vi "Manipulate FROG Trace.vi"(8 "error in (no error)":errorcluster caption="entrée d'erreur (pas d'erreur)", 10 "Transpose FROG Trace":bool, 11 "File mainpulate en entrée":refnum<class "File manipulate.lvclass">) -> (0 "error out":errorcluster caption="sortie d'erreur", 1 "Wavelenght_New":dbl[](array[numeric]), 2 "DelayVector":dbl[](array[numeric]), 3 "File mainpulate en sortie":refnum<class "File manipulate.lvclass">, 4 "Data Reshape":dbl[][](array[numeric]), 5 "Data Manipulate FROG TRACE":T1 {"WavelengthPoints_increment" format="%.16f"; "WavelengthPoints_center" format="%#.13g"})   [LabVIEW 2024, in "File manipulate.lvclass"]
uses:
  File manipulate.lvclass
  Data Manipulate FROG TRACE.ctl
  FROG Trace -Etat.ctl
  File manipulate.lvclass/File manipulate.ctl
  <userlib>/_Hooovahh/Array VIMs/Controls/Enum - Rows Columns.ctl
  <vilib>/Analysis/1siggen.llb/Ramp Pattern by Samples.vi
  6a061561-2aec-49c3-b07e-13be07ae40b1.vi
  d13b3189-b418-4897-bbe3-08cafe995864.vi
  <vilib>/Analysis/baseanly.llb/Mean (DBL).vi
  <vilib>/gmath/interp.llb/Interpolate 2D (1d xi,yi).vi
  <vilib>/Analysis/NI_AALBase.lvlib
  <vilib>/gmath/NI_Gmath.lvlib
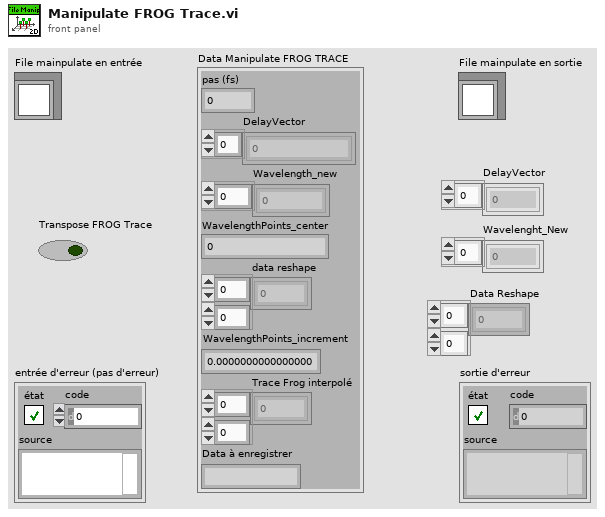
[diagram p1: front panel]
types:
  T1 = typedef "File manipulate.lvclass/Data Manipulate FROG TRACE.ctl" = cluster{"pas (fs)":ext, "DelayVector":dbl[], "Wavelength_new":dbl[], "WavelengthPoints_center":dbl, "data reshape":dbl[][], "WavelengthPoints_increment":dbl, "Trace Frog interpolé":dbl[][], "Data à enregistrer":string}
  T2 = typedef "File manipulate.lvclass/FROG Trace -Etat.ctl" = enum16{"Conversion Pas um to fs", "Delay Vector", "Reshape FROG Trace", "Wavelenght New", "Wavelenght Center", "Wavelenght Point increment", "Interpolation 2D", "Concaner en txt", "Enregistrement"}
  T3 = typedef "Enum - Rows Columns.ctl" = enum16{"Rows", "Columns"}
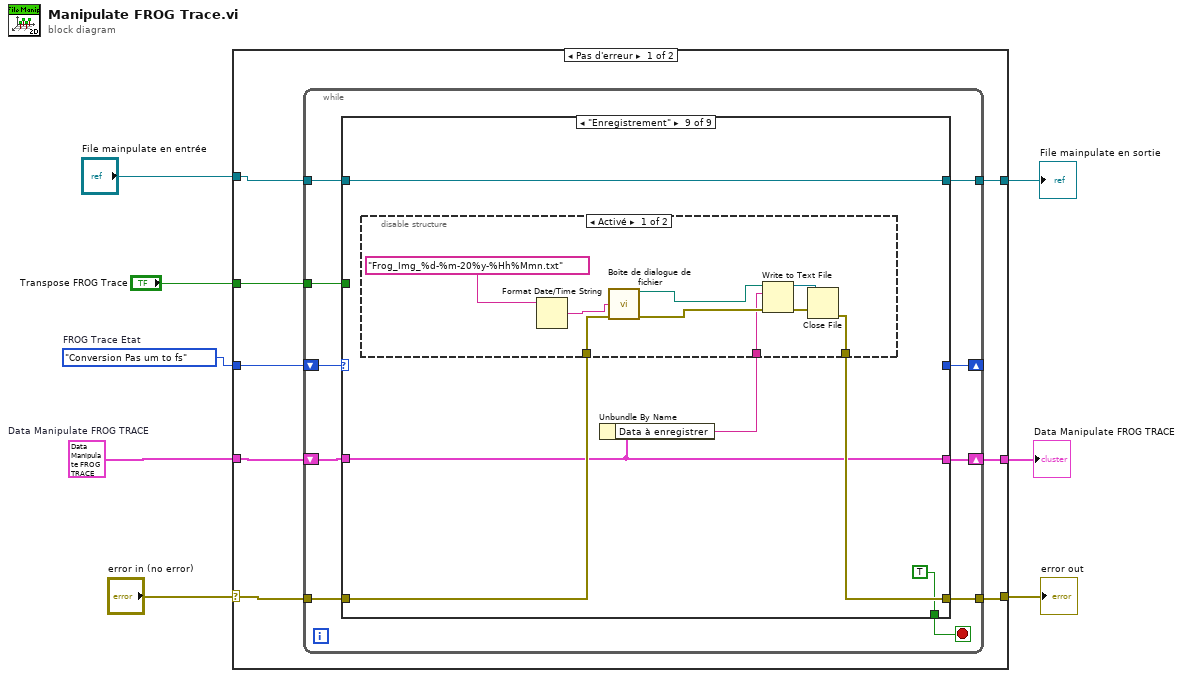
[diagram p0: block diagram]
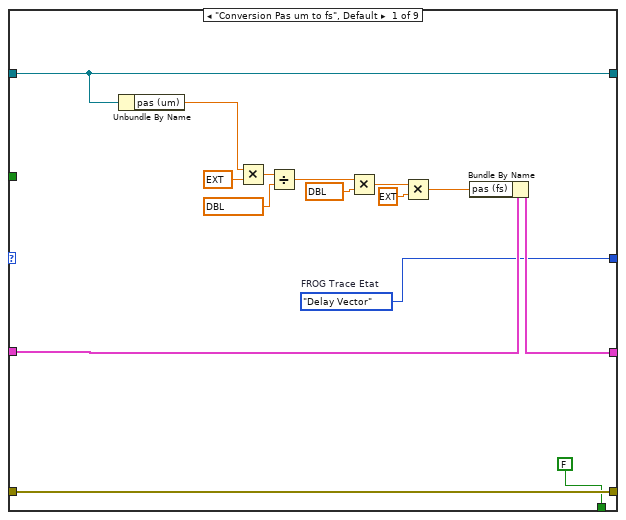
[diagram p2: hidden frame]
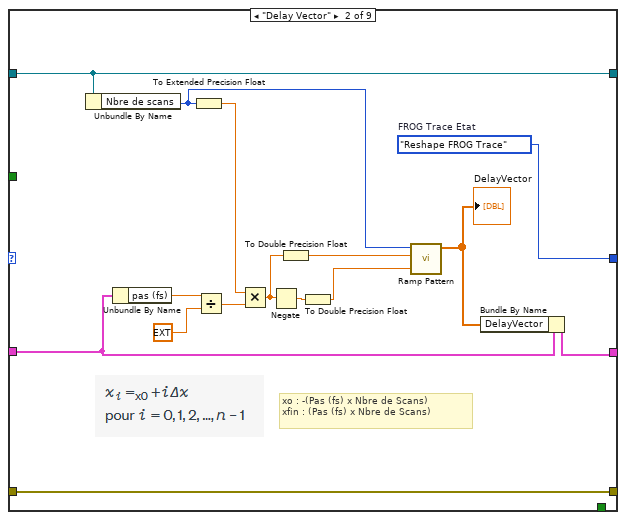
[diagram p3: hidden frame]
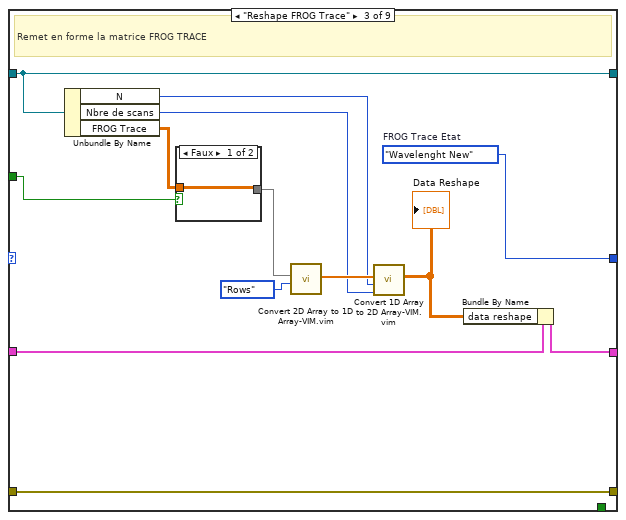
[diagram p4: hidden frame]
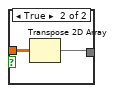
[diagram p5: hidden frame]
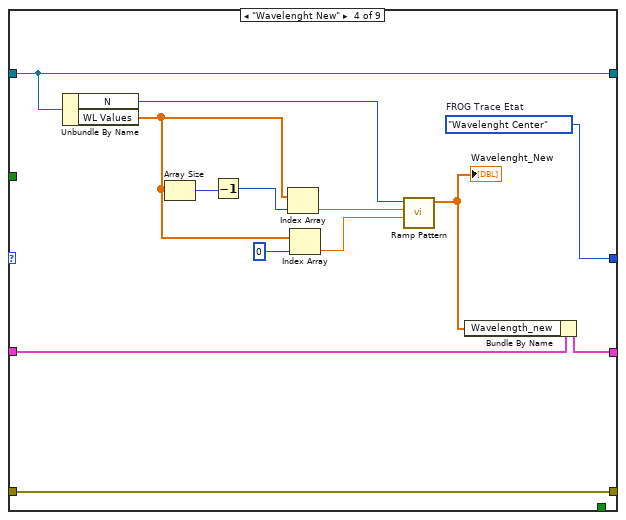
[diagram p6: hidden frame]
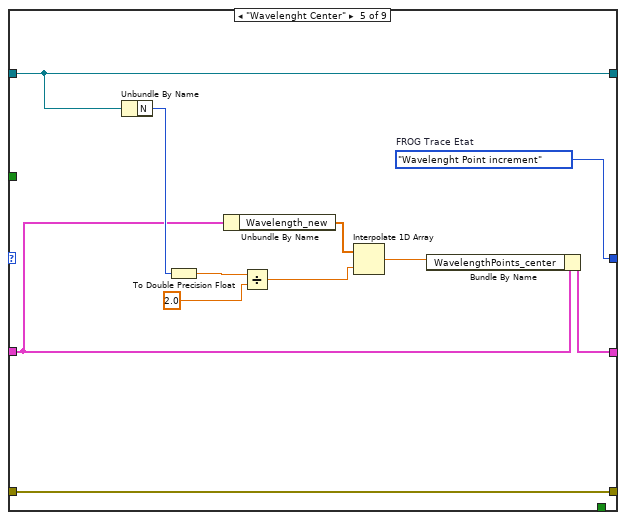
[diagram p7: hidden frame]
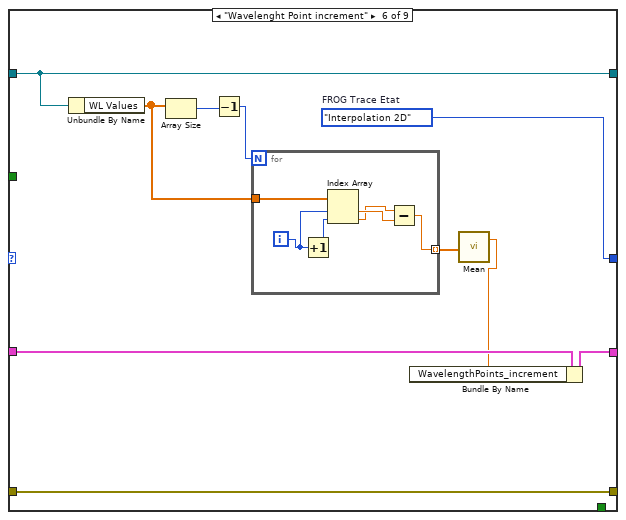
[diagram p8: hidden frame]
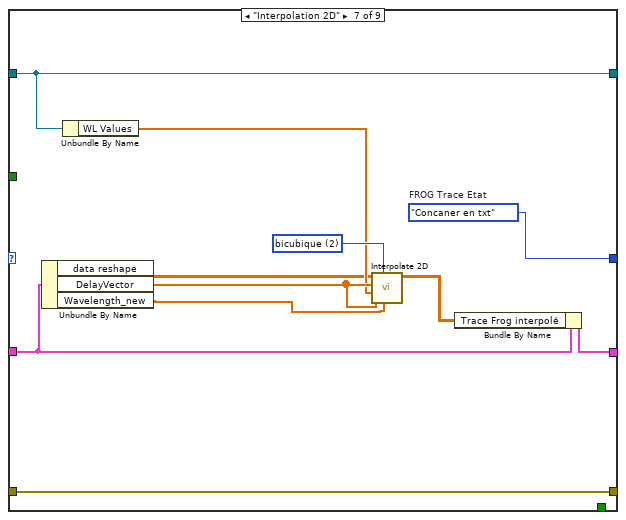
[diagram p9: hidden frame]
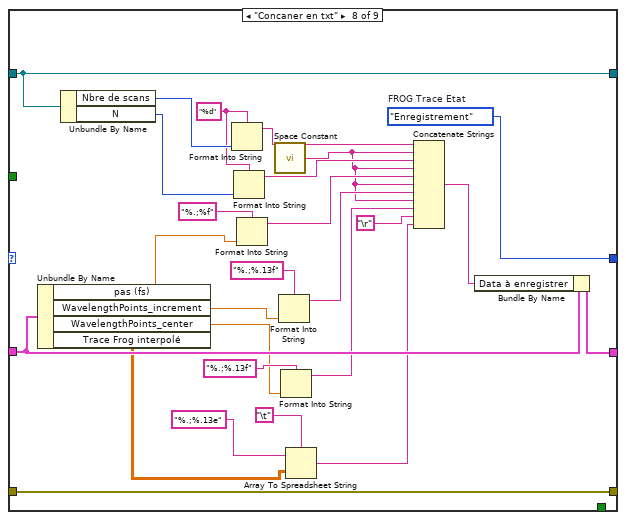
[diagram p10: hidden frame]
diagram:
  w3 = T1 {"pas (fs)"=0.0, "DelayVector"=[], "Wavelength_new"=[], "WavelengthPoints_center"=0.0, "data reshape"=[], "WavelengthPoints_increment"=0.0, "Trace Frog interpolé"=[], "Data à enregistrer"=""}  # Data Manipulate FROG TRACE
  w4 = FROG_Trace_-Etat."Conversion Pas um to fs"  # FROG Trace Etat
  n1 = case shown="Pas d'erreur" "error in (no error)" {
    selector: "error in (no error)" -> [w14 w167]
    tunnel: [w15 w167] -> w7
    tunnel: [w12 w166] -> w5
    tunnel: "File mainpulate en entrée" -> [w13 w166]
    tunnel: w4 -> [w16 _]
    tunnel: w3 -> [w11 w165]
    tunnel: "Transpose FROG Trace" -> [w10 _]
    tunnel: [w9 w165] -> w1
    frame No Error {
      n2 = while {
        shift-right: [w25] -> _
        shift-left: w16 -> [w26]
        tunnel: [w24] -> w15
        tunnel: w14 -> [w23]
        shift-right: [w19] -> w9
        shift-left: w11 -> [w20]
        tunnel: w10 -> [w18]
        tunnel: w13 -> [w21]
        tunnel: [w22] -> w12
        stop <- w17 stop-if-true
        n3 = case shown="\"Enregistrement\"" w26 {
          tunnel: [w28 w42 w57 w73 w86 w97 w122 w125 _] -> w25
          tunnel: [w41 w56 w69 w85 w96 w106 w123 w149 w153] -> w24
          tunnel: w23 -> [w41 w56 w69 w85 w96 w106 w123 w149 w154]
          tunnel: [w33 w55 w67 w83 w92 w104 w118 w148 w155] -> w22
          tunnel: w21 -> [w33 w55 w67 w83 w92 w104 w118 w148 w155]
          tunnel: w20 -> [w31 w54 w68 w84 w90 w105 w120 w143 w152]
          tunnel: [w30 w44 w59 w75 w88 w99 w115 w127 w152] -> w19
          tunnel: w18 -> [_ _ w66 _ _ _ _ _ _]
          tunnel: [FALSE _ _ _ _ _ _ _ TRUE] -> w17
          frame "Conversion Pas um to fs", Default {
            w28 = FROG_Trace_-Etat."Delay Vector"  # FROG Trace Etat
            n4 = Unbundle By Name(w33) -> ("pas (um)"=w32:ext)
            n5 = Multiply(x=w32, y=ext 1e-06) -> (x*y=w36:ext)
            n6 = Divide(x=w36, y=ext[unit] 300000000.0) -> (x/y=w40:ext[unit])
            n7 = Multiply(x=w40, y=ext[unit] 1000000000000000.0) -> (x*y=w35:ext)
            n8 = Multiply(x=w35, y=ext 2.0) -> (x*y=w29:ext)
            n9 = Bundle By Name(cluster=w31, "pas (fs)"=w29) -> (w30:T1)
          }
          frame "Delay Vector" {
            w42 = FROG_Trace_-Etat."Reshape FROG Trace"  # FROG Trace Etat
            # "xo : -(Pas (fs) x Nbre de Scans)\nxfin : (Pas (fs) x Nbre de Scans)"
            n10 = Unbundle By Name(w55) -> ("Nbre de scans"=w45:i32)
            n11 = Unbundle By Name(w54) -> ("pas (fs)"=w53:ext)
            n12 = To Extended Precision Float(1:w45) -> (0:w50:ext)
            n13 = Divide(x=w53, y=ext 2.0) -> (x/y=w51:ext)
            n14 = Multiply(x=w50, y=w51) -> (x*y=w47:ext)
            n15 = Negate(x=w47) -> (-x=w49:ext)
            n16 = To Double Precision Float(number=w47) -> (double precision float=w46:dbl)
            n17 = To Double Precision Float(number=w49) -> (double precision float=w48:dbl)
            n18 = call-poly <vilib>:"Ramp Pattern.vi"("start"=w48, "end"=w46, "samples"=w45) -> ("Ramp Pattern"=w43:dbl[])  [unwired: 7 in, 1 out]
            "DelayVector" <- w43
            n19 = Bundle By Name(cluster=w54, "DelayVector"=w43) -> (w44:T1)
          }
          frame "Reshape FROG Trace" {
            w57 = FROG_Trace_-Etat."Wavelenght New"  # FROG Trace Etat
            # "Remet en forme la matrice FROG TRACE"
            n20 = Unbundle By Name(w67) -> ("N"=w61:i32, "Nbre de scans"=w60:i32, "FROG Trace"=w65:dbl[][])
            n21 = case shown="Faux" w66 {
              tunnel: w65 -> [w70 w72]
              tunnel: [w70 w71] -> w63
              frame False {
              }
              frame True {
                n22 = Transpose 2D Array(2D array=w72) -> (transposed array=w71:dbl[][])
              }
            }
            n23 = call "Convert 2D Array to 1D Array-VIM.vim"("Concatenate (rows)"=Enum_-_Rows_Columns."Rows", "2D Array"=w63) -> ("1D Array"=w62:dbl[])  [unwired: 9 in]
            n24 = call "Convert 1D Array to 2D Array-VIM.vim"("Number of Columns"=w60, "Number of Rows"=w61, "1D Array"=w62) -> ("2D Array"=w58:dbl[][])  [unwired: 8 in]
            "Data Reshape" <- w58
            n25 = Bundle By Name(cluster=w68, "data reshape"=w58) -> (w59:T1)
          }
          frame "Wavelenght New" {
            w73 = FROG_Trace_-Etat."Wavelenght Center"  # FROG Trace Etat
            n26 = Unbundle By Name(w83) -> ("N"=w76:i32, "WL Values"=w79:dbl[])
            n27 = Array Size(array=w79) -> (size(s)=w82:i32)
            n28 = Decrement(x=w82) -> (x-1=w81:i32)
            n29 = Index Array(array=w79, index=w81) -> (element=w80:dbl)
            n30 = Index Array(array=w79, index=0 ("indice")) -> (element=w77:dbl)
            n31 = call-poly <vilib>:"Ramp Pattern.vi"("start"=w77, "end"=w80, "samples"=w76) -> ("Ramp Pattern"=w74:dbl[])  [unwired: 7 in, 1 out]
            "Wavelenght_New" <- w74
            n32 = Bundle By Name(cluster=w84, "Wavelength_new"=w74) -> (w75:T1)
          }
          frame "Wavelenght Center" {
            w86 = FROG_Trace_-Etat."Wavelenght Point increment"  # FROG Trace Etat
            n33 = Unbundle By Name(w92) -> ("N"=w91:i32)
            n34 = To Double Precision Float(number=w91) -> (double precision float=w95:dbl)
            n35 = Unbundle By Name(w90) -> ("Wavelength_new"=w89:dbl[])
            n36 = Divide(x=w95, y=2.0) -> (x/y=w94:dbl)
            n37 = Interpolate 1D Array(1:w94, 2:w89) -> (0:w87:dbl)
            n38 = Bundle By Name(cluster=w90, "WavelengthPoints_center"=w87) -> (w88:T1)
          }
          frame "Wavelenght Point increment" {
            w97 = FROG_Trace_-Etat."Interpolation 2D"  # FROG Trace Etat
            n39 = Unbundle By Name(w104) -> ("WL Values"=w102:dbl[])
            n40 = Array Size(array=w102) -> (size(s)=w103:i32)
            n41 = Decrement(x=w103) -> (x-1=w101:i32)
            n42 = for {
              N: w101 -> [_]
              tunnel: [w110] -> w100 mode=indexing
              tunnel: w102 -> [w108]
              i -> [w111]
              n43 = Increment(x=w111) -> (x+1=w112:i32)
              n44 = Index Array(array=w108, index #1=w111, index #2=w112) -> (element #1=w109:dbl, element #2=w107:dbl)
              n45 = Subtract(x=w107, y=w109) -> (x-y=w110:dbl)
            }
            n46 = call-poly <vilib>:"Mean.vi"("X"=w100) -> ("mean"=w98:dbl)  [unwired: 1 out]
            n47 = Bundle By Name(cluster=w105, "WavelengthPoints_increment"=w98) -> (w99:T1)
          }
          frame "Interpolation 2D" {
            w121 = 2 items=["plus proche voisin", "bilinéaire", "bicubique", "spline bicubique"] ("method")
            w122 = FROG_Trace_-Etat."Concaner en txt"  # FROG Trace Etat
            n48 = Unbundle By Name(w120) -> ("data reshape"=w116:dbl[][], "DelayVector"=w119:dbl[], "Wavelength_new"=w113:dbl[])
            n49 = Unbundle By Name(w118) -> ("WL Values"=w117:dbl[])
            n50 = call-poly <vilib>:"Interpolate 2D.vi"("yi"=w113, "method"=w121, "xi"=w119, "Y"=w117, "X"=w119, "Z"=w116) -> ("zi"=w114:dbl[][])  [unwired: 2 in, 3 out]
            n51 = Bundle By Name(cluster=w120, "Trace Frog interpolé"=w114) -> (w115:T1)
          }
          frame "Concaner en txt" {
            w125 = FROG_Trace_-Etat."Enregistrement"  # FROG Trace Etat
            w124 = "%d" ("chaîne de format")
            n52 = Unbundle By Name(w143) -> ("pas (fs)"=w141:ext, "WavelengthPoints_increment"=w138:dbl, "WavelengthPoints_center"=w134:dbl, "Trace Frog interpolé"=w129:dbl[][])
            n53 = Unbundle By Name(w148) -> ("Nbre de scans"=w147:i32, "N"=w145:i32)
            n54 = Format Into String(format string=w124, w147) -> (resulting string=w146:string)  [unwired: 2 in, 1 out]
            n55 = Format Into String(format string=w124, w145) -> (resulting string=w144:string)  [unwired: 2 in, 1 out]
            n56 = Format Into String(format string="%.;%f" ("chaîne de format"), w141) -> (resulting string=w140:string)  [unwired: 2 in, 1 out]
            n57 = call <vilib>:"Space Constant.vi"() -> ("String"=w136:string)
            n58 = Format Into String(format string="%.;%.13f" ("chaîne de format"), w138) -> (resulting string=w137:string)  [unwired: 2 in, 1 out]
            n59 = Format Into String(format string="%.;%.13f" ("chaîne de format"), w134) -> (resulting string=w133:string)  [unwired: 2 in, 1 out]
            n60 = Array To Spreadsheet String(delimiter (Tab)="\t", array=w129, 3:"%.;%.13e" ("chaîne de format")) -> (spreadsheet string=w128:string)
            n61 = Concatenate Strings(w146, w136, w144, w136, w140, w136, w137, w136, w133, "\r", w128) -> (w126:string)
            n62 = Bundle By Name(cluster=w143, "Data à enregistrer"=w126) -> (w127:T1)
          }
          frame "Enregistrement" {
            n63 = Unbundle By Name(w152) -> ("Data à enregistrer"=w151:string)
            n64 = disable-structure shown="Activé" {
              disable-tunnel: w154 -> [w158 _]
              disable-tunnel: [w157 _] -> w153
              disable-tunnel: w151 -> [w156 _]
              frame Enabled {
                n65 = Format Date/Time String(time format string (%c)="Frog_Img_%d-%m-20%y-%Hh%Mmn.txt") -> (date/time string=w159:string)  [unwired: 2 out]
                n66 = call "Boîte de dialogue de fichier"("default name"=w159, "error in"=w158) -> ("selected path"=w163:path, "error out"=w161:errorcluster)  [unwired: 10 in, 2 out]
                n67 = Write to Text File(file (use dialog)=w163, text=w156, error in=w161) -> (refnum out=w162:refnum<file>, error out=w160:errorcluster)  [unwired: 1 in, 1 out]
                n68 = Close File(refnum=w162, error in=w160) -> (error out=w157:errorcluster)  [unwired: 1 out]
              }
              frame Disabled {
              }
            }
          }
        }
      }
    }
    frame Error {
    }
  }
  "error out" <- w7
  "File mainpulate en sortie" <- w5
  "Data Manipulate FROG TRACE" <- w1
